vi "Keithley 2002 Calc2 Config.vi"(1 "error in":T1, 2 "calculation1 (none:5)":u16(ring)=5 items=["mean", "standard deviation", "maximum", "mimimum", "peak-to-peak", "none"], 3 "GPIB address":string="16") -> (0 "error out":T1)   [LabVIEW 2020]
doc: "This VI is used to configure the settings for math calculation 2. This involves operations on readings stored in the buffer.\n\nTo read the results of the calculation, use the Calc Read VI."
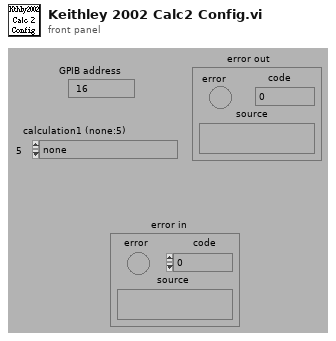
[diagram p1: front panel]
types:
  T1 = cluster{"error":bool, "code":i32, "source":string}
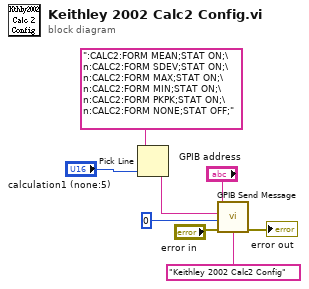
[diagram p0: block diagram]
diagram:
  n1 = Pick Line(multi-line string=":CALC2:FORM MEAN;STAT ON;\n:CALC2:FORM SDEV;STAT ON;\n:CALC2:FORM MAX;STAT ON;\n:CALC2:FORM MIN;STAT ON;\n:CALC2:FORM PKPK;STAT ON;\n:CALC2:FORM NONE;STAT OFF;", line index="calculation1 (none:5)") -> (output string=w1:string)  [unwired: 1 in]
  n2 = call "GPIB Send Message.vi"("address string"="GPIB address", "write buffer"=w1, "source"="Keithley 2002 Calc2 Config", "write mode (set END:0)"=0, "error in"="error in") -> ("error out"=→"error out":T1)  [unwired: 2 in, 2 out]
